vi "DataVIS_Read .DAT Data.vi"(8 "error in (no error)":errorcluster, 11 "file path (use dialog)":path) -> (0 "error out":errorcluster, 3 "all stacked channels":dbl[](array[numeric]))   [LabVIEW 2016]
panel:
  out "Waveform Graph":dbl[](graph)
  out "data":cluster{"all stacked channels":dbl[]}[](array[cluster])
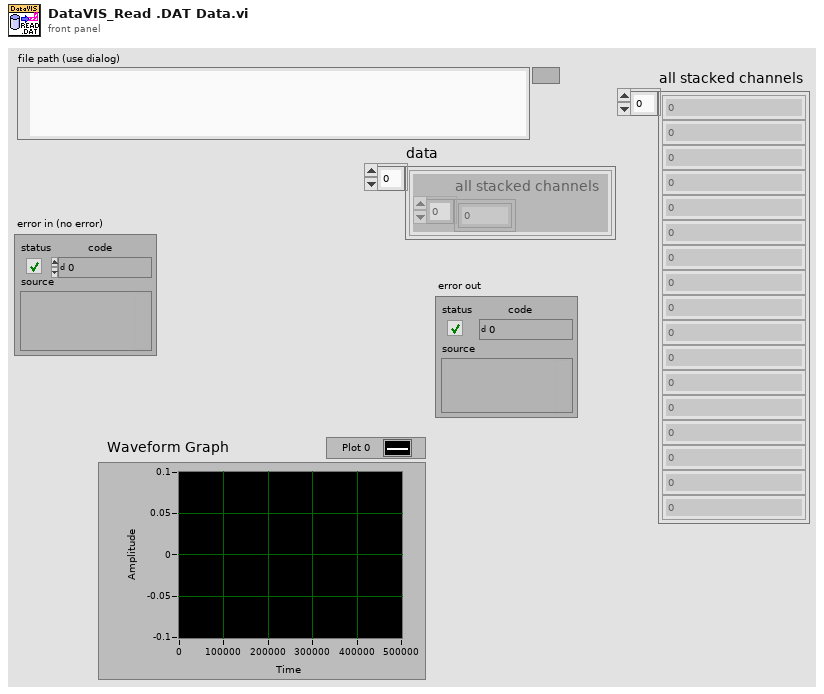
[diagram p1: front panel]
types:
  T1 = enum16{"open", "replace", "create", "open or create", "replace or create", "replace or create with confirmation"}
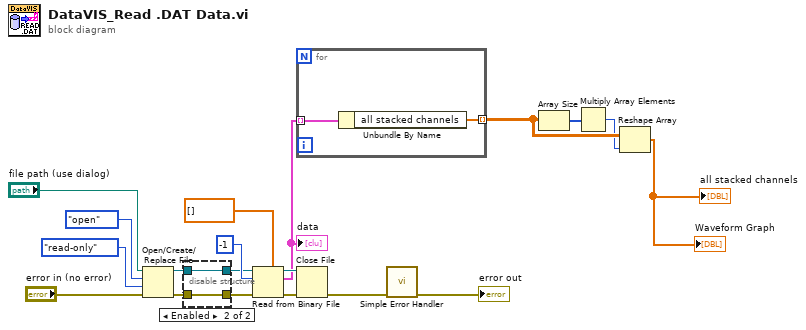
[diagram p0: block diagram]
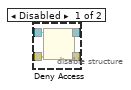
[diagram p2: hidden frame]
diagram:
  n1 = Open/Create/Replace File(file path (use dialog)="file path (use dialog)", error in="error in (no error)", operation (0:open)=T1."open", access (0:read/write)=enum16{"read/write", "read-only", "write-only"}."read-only") -> (refnum out=w16:refnum<file>, error out=w15:errorcluster)  [unwired: 2 in, 1 out]
  n2 = disable-structure shown="Enabled" {
    disable-tunnel: w16 -> [w23 w25]
    disable-tunnel: w15 -> [w22 w24]
    disable-tunnel: [w21 w24] -> w7
    disable-tunnel: [w20 w25] -> w6
    frame Disabled {
      n3 = Deny Access(4:w22, 7:w23) -> (0:w21:errorcluster, 3:w20:refnum<file>)  [unwired: 1 in]
    }
    frame Enabled {
    }
  }
  n4 = Read from Binary File(5:dbl[] [] ("all stacked channels"), 8:w7, 10:-1 ("count (1)"), 11:w6) -> (0:w12:errorcluster, 2:w5:cluster{"all stacked channels":dbl[]}[], 3:w11:refnum<file>)  [unwired: 2 in, 1 out]
  "data" <- w5
  n5 = for {
    tunnel: w5 -> [w27] mode=indexing
    tunnel: [w26] -> w4 mode=indexing
    n6 = Unbundle By Name(w27) -> ("all stacked channels"=w26:dbl[])
  }
  n7 = Close File(refnum=w11, error in=w12) -> (error out=w13:errorcluster)  [unwired: 1 out]
  n8 = call <vilib>:"Simple Error Handler.vi"("error in (no error)"=w13) -> ("error out"=→"error out":errorcluster)  [unwired: 4 in, 4 out]
  n9 = Array Size(array=w4) -> (size(s)=w3:i32[])
  n10 = Multiply Array Elements(1:w3) -> (0:w2:i32)
  n11 = Reshape Array(w4, w2) -> (→"all stacked channels" →"Waveform Graph":dbl[])
